vi "Disable Markers.vi"(8 "error in (no error)":errorcluster, 11 "VISA resource name":refnum<visa-resource-name>) -> (0 "error out":errorcluster, 3 "VISA resource name out":refnum<visa-resource-name>)   [LabVIEW 2009, in "Agilent PSG MXG Series.lvlib"]
doc: "Turns off all active markers.\n\n<B>Notes:</B>\n(1) This VI is valid only in E8247C, E8257C, E8267C, E8257D, E8267D that install <B>Option 007</B> (Analog ramp sweep) and N5183A."
uses:
  Agilent PSG MXG Series.lvlib
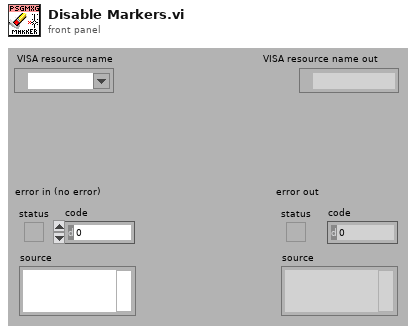
[diagram p1: front panel]
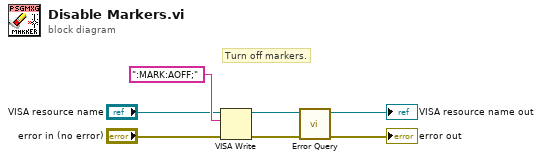
[diagram p0: block diagram]
diagram:
  # "Turn off markers."
  n1 = VISA Write(VISA resource name="VISA resource name", write buffer=":MARK:AOFF;", error in (no error)="error in (no error)") -> (VISA resource name out=w7:refnum<visa-resource-name>, error out=w6:errorcluster)  [unwired: 1 out]
  n2 = call "Error Query.vi"("error in (no error)"=w6, "VISA resource name"=w7) -> ("error out"=→"error out":errorcluster, "VISA resource name out"=→"VISA resource name out":refnum<visa-resource-name>)  [unwired: 8 out]
